vi "XML To Data.vi"(1 "XML Data":string, 2 "Name":string) -> ()   [LabVIEW 2013]
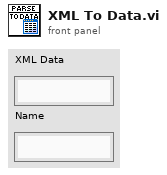
[diagram p1: front panel]
types:
  T1 = typedef "Semaphore RefNum" = refnum<k1>
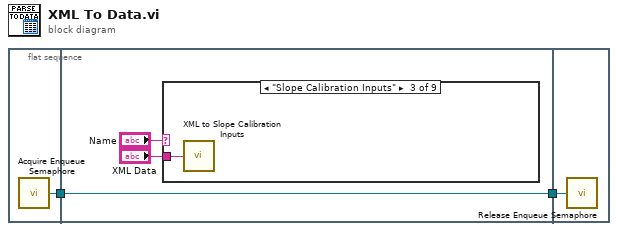
[diagram p0: block diagram]
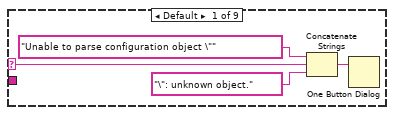
[diagram p2: hidden frame]
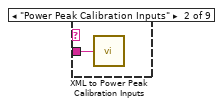
[diagram p3: hidden frame]
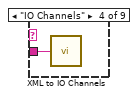
[diagram p4: hidden frame]
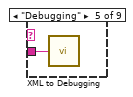
[diagram p5: hidden frame]
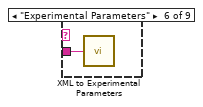
[diagram p6: hidden frame]
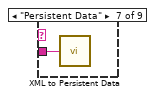
[diagram p7: hidden frame]
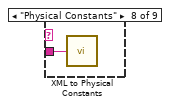
[diagram p8: hidden frame]
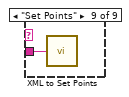
[diagram p9: hidden frame]
diagram:
  n1 = flat-sequence {
    tunnel: [w3] -> w1
    tunnel: [w4] -> w2
    tunnel: w1 -> [w4]
    tunnel: w2 -> [w19]
    frame #0 {
      n2 = call "Acquire Enqueue Semaphore.vi"() -> ("Semaphore Reference"=w3:T1)
    }
    frame #1 {
      n3 = case shown="\"Slope Calibration Inputs\"" "Name" {
        selector: "Name" -> [w8 _ _ _ _ _ _ _ _]
        tunnel: "XML Data" -> [_ w11 w12 w13 w14 w15 w16 w17 w18]
        frame Default {
          n4 = Concatenate Strings("Unable to parse configuration object \"" ("string"), w8, "\": unknown object." ("string")) -> (w9:string)
          n5 = One Button Dialog(message=w9) -> ()  [unwired: 1 in, 1 out]
        }
        frame "Power Peak Calibration Inputs" {
          n6 = call "XML to Power Peak Calibration Inputs.vi"("XML Data"=w11) -> ()
        }
        frame "Slope Calibration Inputs" {
          n7 = call "XML to Slope Calibration Inputs.vi"("XML Data"=w12) -> ()
        }
        frame "IO Channels" {
          n8 = call "XML to IO Channels.vi"("XML Data"=w13) -> ()
        }
        frame "Debugging" {
          n9 = call "XML to Debugging.vi"("XML Data"=w14) -> ()
        }
        frame "Experimental Parameters" {
          n10 = call "XML to Experimental Parameters.vi"("XML Data"=w15) -> ()
        }
        frame "Persistent Data" {
          n11 = call "XML to Persistent Data.vi"("XML Data"=w16) -> ()
        }
        frame "Physical Constants" {
          n12 = call "XML to Physical Constants.vi"("XML Data"=w17) -> ()
        }
        frame "Set Points" {
          n13 = call "XML to Set Points.vi"("XML Data"=w18) -> ()
        }
      }
    }
    frame #2 {
      n14 = call "Release Enqueue Semaphore.vi"("Semaphore Reference"=w19) -> ()
    }
  }
